vi "Filter Get Threshold.vi"(11 "threshold":sgl) -> (2 "function return":u32, 3 "threshold out":sgl)   [LabVIEW 2018, in "AndorSDK.lvlib"]
doc: "EXPNETTYPE unsigned int WINAPI Filter_GetThreshold(float * threshold);"
uses:
  AndorSDK.lvlib
  ATMCD32D.dll
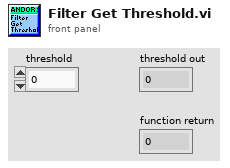
[diagram p1: front panel]
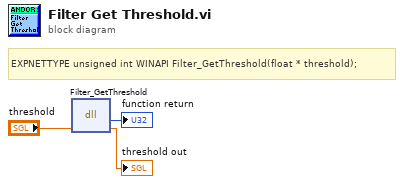
[diagram p0: block diagram]
diagram:
  # "EXPNETTYPE unsigned int WINAPI Filter_GetThreshold(float * threshold);"
  n1 = dll-call lib="PTH2babs E\nPersönliches02 - Arbeit03-HiwijobsLabviewCodelibANDOR\tAndor SDK\nATMCD32D.*" fn="Filter_GetThreshold"("threshold"="threshold") -> (→"function return":u32, "threshold"=→"threshold out":sgl)  [unwired: 3 in, 2 out]
